vi "WordRp.vi"(0 "Type":string="JMS", 1 "Date":string="2015/12/7-14:16", 2 "Grade":string="Admin", 3 "data":dbl[][](array[numeric])=[[0.0, 0.0, 1.0, -14.1]] format="%#.2g", 4 "row headers":string[](array[string])=["ID", "Class", "Num", "Angle "], 5 "error in (no error)":errorcluster caption="错误输入（无错误）", 6 "Operator":string="俞忠达") -> (14 "添加的路径":path=path "C:/Users/jms/Desktop/MEMS WIN8/MEMS WIN8/Data Base/Blade Test Report.docx", 19 "error out":errorcluster={"status"=TRUE, "code"=7, "source"="NI_Word.lvclass:new report subVI.vi -> NI_report.lvclass:New Report.vi -> WordRp.vi -> DB_Main.vi\r\n"} caption="错误输出")   [LabVIEW 2016]
uses:
  <vilib>/Utility/NIReport.llb/Append Report Text (str wrap).vi
  <vilib>/addons/_office/word.llb/Word Easy Table (num).vi
  Controls/Global.vi
  <vilib>/Utility/NIReport.llb/NI_report.lvclass
  <vilib>/addons/_office/NI_ReportGenerationToolkit.lvlib
  <vilib>/Utility/NIReport.llb/Word/NI_Word.lvclass
  <vilib>/Analysis/NI_AALBase.lvlib
panel:
  in  "路径":path=path "C:/Users/jms/Desktop/MEMS WIN8/MEMS WIN8/Blade Test Report.docx"
  in  "axis font 2":T1={"font style"="", "bold"=FALSE, "italic"=TRUE, "underline"=FALSE, "size"=8.0, "color"=0}
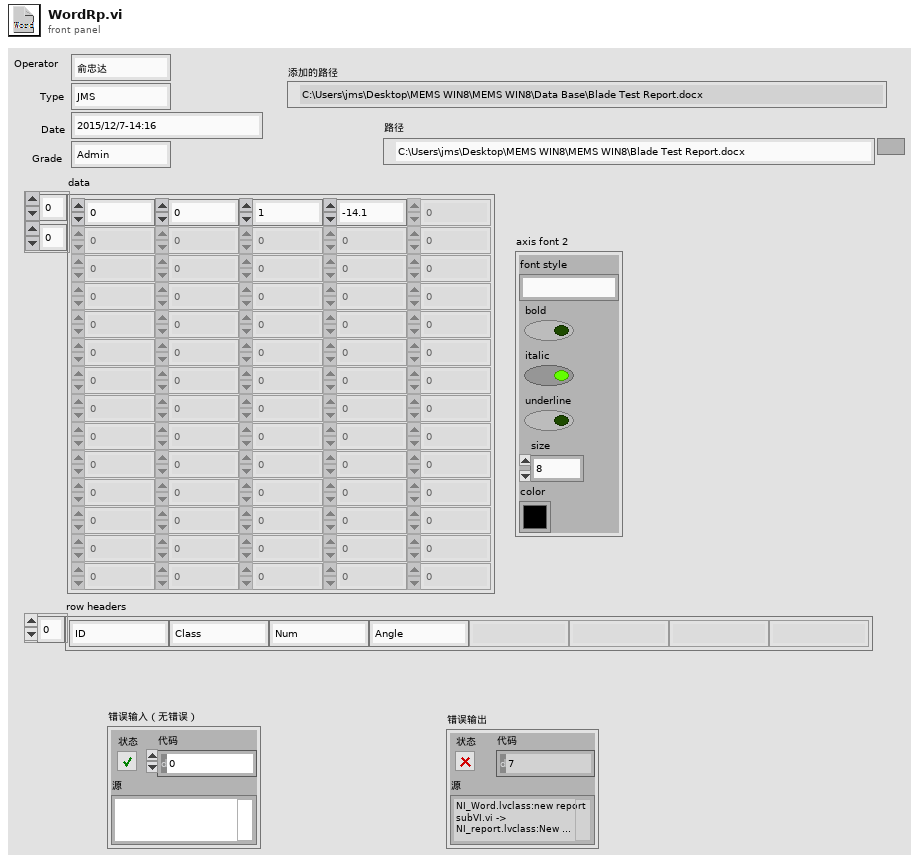
[diagram p1: front panel]
types:
  T1 = cluster{"font style":string, "bold":bool, "italic":bool, "underline":bool, "size":sgl, "color":u32}
  T2 = cluster{"position (excel)":cluster{"row":i32, "column":i32}, "name (excel)":string, "bookmark (word)":string}
  T3 = enum16{"Standard Report", "HTML", "Word", "Excel"}
  T4 = enum32{"invalid app kind", "Development System", "Run Time System", "Student Edition", "Embedded LabVIEW", "Evaluation", "Custom"}
  T5 = cluster{"Alignment":enum16{"Left", "Centered", "Right", "Justify"}, "Left":dbl, "Right":dbl, "Special":enum16{"(none)", "First line", "Hanging"}, "By":dbl, "Before":dbl, "After":dbl, "Line spacing":enum16{"Single", "1,5 lines", "Double", "At least", "Exactly", "Multiple"}, "At":dbl}
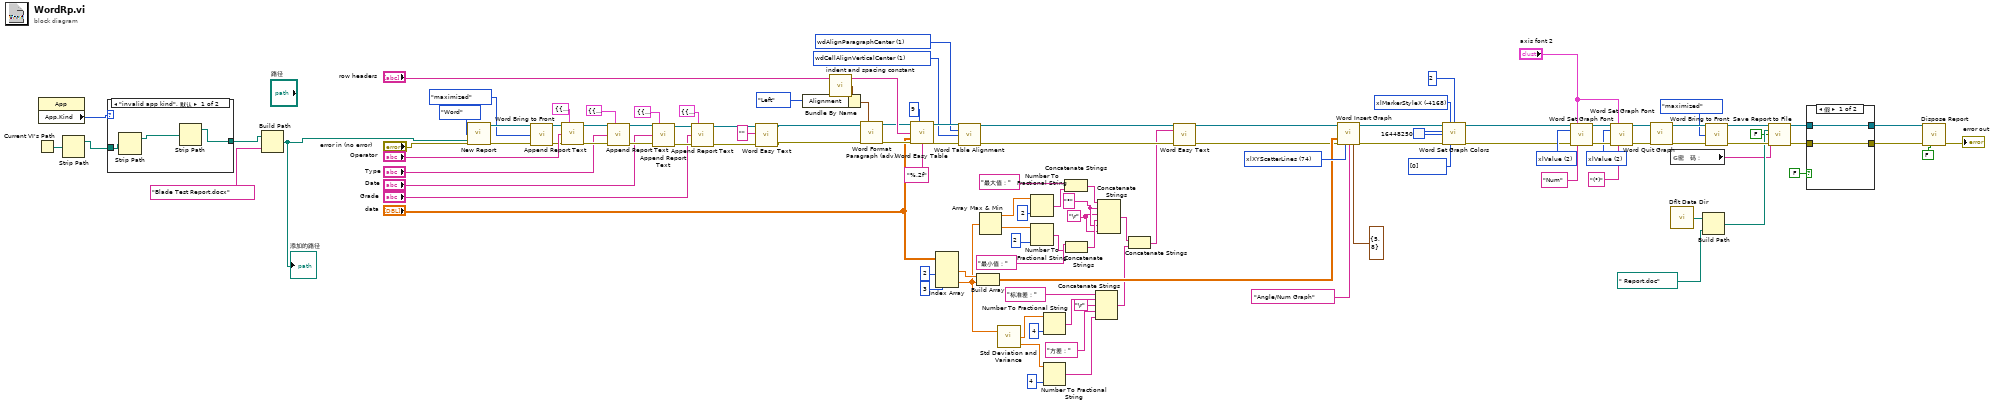
[diagram p0: block diagram]
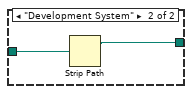
[diagram p2: hidden frame]
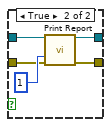
[diagram p3: hidden frame]
diagram:
  w36 = "°" ("字符串")
  w21 = "\r"
  w59 = 2 items=["xlCategory"=1, "xlSeriesAxis"=3, "xlValue"=2] ("axis type")
  w62 = 2 items=["xlCategory"=1, "xlSeriesAxis"=3, "xlValue"=2] ("axis type")
  w66 = u32 16448250 ("plot area color")
  w67 = -4168 items=["xlMarkerStyleAutomatic"=-4105, "xlMarkerStyleCircle"=8, "xlMarkerStyleDash"=-4115, "xlMarkerStyleDiamond"=2, "xlMarkerStyleDot"=-4118, "xlMarkerStyleNone"=-4142, "xlMarkerStylePicture"=-4147, "xlMarkerStylePlus"=9, "xlMarkerStyleSquare"=1, "xlMarkerStyleStar"=5, "xlMarkerStyleTriangle"=3, "xlMarkerStyleX"=-4168] ("marker style")
  w73 = 1 items=["wdAlignParagraphLeft"=0, "wdAlignParagraphCenter"=1, "wdAlignParagraphRight"=2, "wdAlignParagraphJustify"=3, "wdAlignParagraphDistribute"=4, "wdAlignParagraphJustifyMed"=5, "wdAlignParagraphJustifyHi"=7, "wdAlignParagraphJustifyLow"=8] ("horizontal alignment")
  w74 = 1 items=["wdCellAlignVerticalTop"=0, "wdCellAlignVerticalCenter"=1, "wdCellAlignVerticalBottom"=3] ("vertical alignment")
  w87 = 74 items=["xlColumnClustered"=51, "xlColumnStacked"=52, "xlColumnStacked100"=53, "xl3DColumnClustered"=54, "xl3DColumnStacked"=55, "xl3DColumnStacked100"=56, "xlBarClustered"=57, "xlBarStacked"=58, "xlBarStacked100"=59, "xl3DBarClustered"=60, "xl3DBarStacked"=61, "xl3DBarStacked100"=62, "xlLineStacked"=63, "xlLineStacked100"=64, "xlLineMarkers"=65, "xlLineMarkersStacked"=66, "xlLineMarkersStacked100"=67, "xlPieOfPie"=68, "xlPieExploded"=69, "xl3DPieExploded"=70, "xlBarOfPie"=71, "xlXYScatterSmooth"=72, "xlXYScatterSmoothNoMarkers"=73, "xlXYScatterLines"=74, "xlXYScatterLinesNoMarkers"=75, "xlAreaStacked"=76, "xlAreaStacked100"=77, "xl3DAreaStacked"=78, "xl3DAreaStacked100"=79, "xlDoughnutExploded"=80, "xlRadarMarkers"=81, "xlRadarFilled"=82, "xlSurface"=83, "xlSurfaceWireframe"=84, "xlSurfaceTopView"=85, "xlSurfaceTopViewWireframe"=86, "xlBubble"=15, "xlBubble3DEffect"=87, "xlStockHLC"=88, "xlStockOHLC"=89, "xlStockVHLC"=90, "xlStockVOHLC"=91, "xlCylinderColClustered"=92, "xlCylinderColStacked"=93, "xlCylinderColStacked100"=94, "xlCylinderBarClustered"=95, "xlCylinderBarStacked"=96, "xlCylinderBarStacked100"=97, "xlCylinderCol"=98, "xlConeColClustered"=99, "xlConeColStacked"=100, "xlConeColStacked100"=101, "xlConeBarClustered"=102, "xlConeBarStacked"=103, "xlConeBarStacked100"=104, "xlConeCol"=105, "xlPyramidColClustered"=106, "xlPyramidColStacked"=107, "xlPyramidColStacked100"=108, "xlPyramidBarClustered"=109, "xlPyramidBarStacked"=110, "xlPyramidBarStacked100"=111, "xlPyramidCol"=112, "xl3DColumn"=-4100, "xlLine"=4, "xl3DLine"=-4101, "xl3DPie"=-4102, "xlPie"=5, "xlXYScatter"=-4169, "xl3DArea"=-4098, "xlArea"=1, "xlDoughnut"=-4120, "xlRadar"=-4151] ("chart type")
  n1 = Current VI's Path() -> (path=w8:path)
  n2 = property class="App"() -> ("App.Kind"=w4:T4)  [unwired: 2 in, 2 out]
  n3 = Strip Path(path=w8) -> (stripped path=w3:path)  [unwired: 1 out]
  n4 = case shown="\"invalid app kind\", 默认" w4 {
    tunnel: w3 -> [w117 w120]
    tunnel: [w118 w119] -> w2
    frame "invalid app kind", Default {
      n5 = Strip Path(path=w117) -> (stripped path=w116:path)  [unwired: 1 out]
      n6 = Strip Path(path=w116) -> (stripped path=w118:path)  [unwired: 1 out]
    }
    frame "Development System" {
      n7 = Strip Path(path=w120) -> (stripped path=w119:path)  [unwired: 1 out]
    }
  }
  n8 = Build Path(base path=w2, name or relative path="Blade Test Report.docx" ("名称或相对路径")) -> (appended path=w5:path)
  "添加的路径" <- w5
  n9 = call <vilib>:"New Report.vi"("report type"=T3."Word", "template (empty)"=w5, "error in (no error)"="error in (no error)") -> ("report out"=w81:refnum<class "NI_report.lvclass">, "error out"=w80:errorcluster)  [unwired: 11 in]
  n10 = call <vilib>:"Word Bring to Front.vi"("report in"=w81, "window state (maximized)"=enum16{"maximized", "minimized", "normal"}."maximized", "error in (no error)"=w80) -> ("report out"=w79:refnum<class "NI_report.lvclass">, "error out"=w78:errorcluster)  [unwired: 11 in]
  n11 = call-poly <vilib>:"Append Report Text.vi"("report in"=w79, "MS Office parameters"=T2 {"position (excel)"={"row"=0, "column"=0}, "name (excel)"="", "bookmark (word)"="Operator"}, "text"="Operator", "error in (no error)"=w78) -> ("report out"=w111:refnum<class "NI_report.lvclass">, "error out"=w109:errorcluster)  [unwired: 8 in, 2 out]
  n12 = call-poly <vilib>:"Append Report Text.vi"("report in"=w111, "MS Office parameters"=T2 {"position (excel)"={"row"=0, "column"=0}, "name (excel)"="", "bookmark (word)"="Type"}, "text"="Type", "error in (no error)"=w109) -> ("report out"=w110:refnum<class "NI_report.lvclass">, "error out"=w108:errorcluster)  [unwired: 8 in, 2 out]
  n13 = call-poly <vilib>:"Append Report Text.vi"("report in"=w110, "MS Office parameters"=T2 {"position (excel)"={"row"=0, "column"=0}, "name (excel)"="", "bookmark (word)"="Date"}, "text"="Date", "error in (no error)"=w108) -> ("report out"=w105:refnum<class "NI_report.lvclass">, "error out"=w104:errorcluster)  [unwired: 8 in, 2 out]
  n14 = call-poly <vilib>:"Append Report Text.vi"("report in"=w105, "MS Office parameters"=T2 {"position (excel)"={"row"=0, "column"=0}, "name (excel)"="", "bookmark (word)"="Grade"}, "text"="Grade", "error in (no error)"=w104) -> ("report out"=w97:refnum<class "NI_report.lvclass">, "error out"=w96:errorcluster)  [unwired: 8 in, 2 out]
  n15 = call <vilib>:"Word Easy Text.vi"("report in"=w97, "text"="", "error in (no error)"=w96) -> ("report out"=w91:refnum<class "NI_report.lvclass">, "error out"=w90:errorcluster)  [unwired: 10 in, 1 out]
  n16 = call <vilib>:"indent and spacing constant.vi"() -> ("indent and spacing"=w94:T5)
  n17 = Bundle By Name(cluster=w94, "Alignment"=enum16{"Left", "Centered", "Right", "Justify"}."Left" ("alignment (left) 2")) -> (w92:T5)
  n18 = call <vilib>:"Word Format Paragraph (adv).vi"("report in"=w91, "indent and spacing"=w92, "error in (no error)"=w90) -> ("report out"=w88:refnum<class "NI_report.lvclass">, "error out"=w89:errorcluster)  [unwired: 4 in, 7 out]
  n19 = call-poly <vilib>:"Word Easy Table.vi"("report in"=w88, "auto format (none)"=9, "column headers"="row headers", "text data"="data", "error in (no error)"=w89, "format string (%.3f)"="%.2f") -> ("report out"=w76:refnum<class "NI_report.lvclass">, "error out"=w75:errorcluster)  [unwired: 7 in, 1 out]
  n20 = Index Array(array="data", index (col) #1=2 ("禁用的索引 (列)"), index (col) #2=3 ("索引 (列)")) -> (element #1=w83:dbl[], element #2=w34:dbl[])  [unwired: 2 in]
  n21 = call <vilib>:"Word Table Alignment.vi"("report in"=w76, "horizontal alignment (left)"=w73, "vertical alignment (top)"=w74, "error in (no error)"=w75) -> ("report out"=w39:refnum<class "NI_report.lvclass">, "error out"=w38:errorcluster)  [unwired: 10 in]
  n22 = Build Array(w83, w34) -> (w72:dbl[][])
  n23 = Array Max & Min(array=w34) -> (max value=w49:dbl, min value=w47:dbl)  [unwired: 2 out]
  n24 = call <vilib>:"Std Deviation and Variance.vi"("X"=w34) -> ("standard deviation"=w33:dbl, "variance"=w28:dbl)  [unwired: 1 in, 1 out]
  n25 = Number To Fractional String(number=w49, precision (6)=i16 2 ("精度(6)")) -> (F-format string=w44:string)  [unwired: 2 in]
  n26 = Number To Fractional String(number=w47, precision (6)=i16 2 ("精度(6)")) -> (F-format string=w42:string)  [unwired: 2 in]
  n27 = Number To Fractional String(number=w33, precision (6)=i16 4 ("精度(6)")) -> (F-format string=w30:string)  [unwired: 2 in]
  n28 = Number To Fractional String(number=w28, precision (6)=i16 4 ("精度(6)")) -> (F-format string=w26:string)  [unwired: 2 in]
  n29 = Concatenate Strings("最大值：", w44) -> (w41:string)
  n30 = Concatenate Strings("最小值：", w42) -> (w40:string)
  n31 = Concatenate Strings("标准差：", w30, "\r", "方差：", w26) -> (w23:string)
  n32 = Concatenate Strings(w41, w36, w21, w40, w36, w21) -> (w24:string)
  n33 = Concatenate Strings(w24, w23) -> (w22:string)
  n34 = call <vilib>:"Word Easy Text.vi"("report in"=w39, "text"=w22, "error in (no error)"=w38) -> ("report out"=w51:refnum<class "NI_report.lvclass">, "error out"=w50:errorcluster)  [unwired: 10 in, 1 out]
  n35 = call <vilib>:"Word Insert Graph.vi"("report in"=w51, "data"=w72, "error in (no error)"=w50, "graph type (col clustered)"=w87, "graph title (\"\")"="Angle/Num Graph" ("graph title (\"\")"), "graph size (5, 5)"=cluster{"height":i32, "width":i32} {"height"=5, "width"=8}) -> ("report out"=w71:refnum<class "NI_report.lvclass">, "error out"=w70:errorcluster)  [unwired: 6 in, 2 out]
  n36 = call <vilib>:"Word Set Graph Colors.vi"("report in"=w71, "marker style (none)"=w67, "weight (1)"=i16 2 ("weight"), "plot area color (w)"=w66, "graph area color (w)"=w66, "error in (no error)"=w70, "plot colors"=u32[] [0]) -> ("report out"=w55:refnum<class "NI_report.lvclass">, "error out"=w56:errorcluster)  [unwired: 7 in]
  n37 = call <vilib>:"Word Set Graph Font.vi"("report in"=w55, "axis font"="axis font 2", "axis type (category)"=w62, "error in (no error)"=w56, "title (\"\")"="Num" ("title (\"\")")) -> ("report out"=w60:refnum<class "NI_report.lvclass">, "error out"=w61:errorcluster)  [unwired: 9 in]
  n38 = call <vilib>:"Word Set Graph Font.vi"("report in"=w60, "axis font"="axis font 2", "axis type (category)"=w59, "error in (no error)"=w61, "title (\"\")"="(°)" ("title (\"\")")) -> ("report out"=w58:refnum<class "NI_report.lvclass">, "error out"=w57:errorcluster)  [unwired: 9 in]
  n39 = call <vilib>:"Word Quit Graph.vi"("report in"=w58, "error in (no error)"=w57) -> ("report out"=w65:refnum<class "NI_report.lvclass">, "error out"=w64:errorcluster)  [unwired: 12 in]
  n40 = global read "Global.vi" "密   码："() -> (w1:string)
  n41 = call <vilib>:"Dflt Data Dir.vi"() -> ("App:Default Data Directory"=w17:path)
  n42 = Build Path(base path=w17, name or relative path=path " Report.doc" ("path")) -> (appended path=w16:path)
  n43 = call <vilib>:"Word Bring to Front.vi"("report in"=w65, "window state (maximized)"=enum16{"maximized", "minimized", "normal"}."maximized", "error in (no error)"=w64) -> ("report out"=w20:refnum<class "NI_report.lvclass">, "error out"=w19:errorcluster)  [unwired: 11 in]
  n44 = call-dynamic "Save Report to File.vi"("report in"=w20, "report file path"=w16, "prompt to replace? (F)"=FALSE, "password (\"\")"=w1, "error in (no error)"=w19) -> ("report out"=w14:refnum<class "NI_report.lvclass">, "error out"=w12:errorcluster)  [unwired: 9 in]
  n45 = case shown="假" FALSE {
    tunnel: w14 -> [w122 w127]
    tunnel: [w122 w126] -> w13
    tunnel: w12 -> [w121 w124]
    tunnel: [w121 w123] -> w11
    frame False {
    }
    frame True {
      n46 = call-dynamic "Print Report.vi"("report in"=w127, "number of copies (1)"=1, "error in (no error)"=w124) -> ("report out"=w126:refnum<class "NI_report.lvclass">, "error out"=w123:errorcluster)  [unwired: 11 in]
    }
  }
  n47 = call-dynamic "Dispose Report.vi"("report in"=w13, "error in (no error)"=w11, "close report? (T)"=FALSE ("Close Report? (T)")) -> ("error out"=→"error out":errorcluster)  [unwired: 12 in]
